vi "XL320_Configure Baud Rate.vi"(8 "error in (no error)":errorcluster, 9 "Baud rate (1,000,000 bps)":T1=3 items=["9600 bps", "57600 bps", "115200 bps", "1,000,000 bps"], 10 "Motor ID (0)":u8, 11 "VISA resource name":refnum<visa-resource-name>) -> (0 "error out":errorcluster, 3 "VISA resource name out":refnum<visa-resource-name>)   [LabVIEW 2017, in "Dynamixel XL320.lvlib"]
doc: "Sets the motor's baud rate. The motor will automatically \"reboot\" and respond to commands sent using the new baud rate."
uses:
  <instrlib>/Dynamixel XL320 (Drivers instrument)/Dynamixel XL320.lvlib
  <instrlib>/Dynamixel XL320 (Drivers instrument)/Public/Motor Operation/Low Level/XL320_Baud Setting.ctl
panel:
  # "Ghislain REMY, IUT de Cachan, 2015 December 2015"
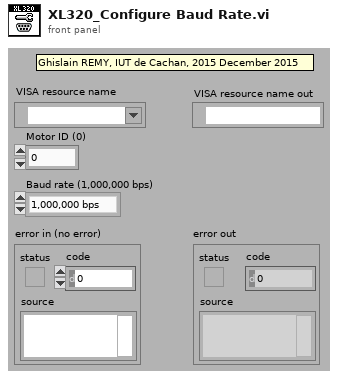
[diagram p1: front panel]
types:
  T1 = typedef "Dynamixel XL320.lvlib/XL320_Baud Setting.ctl" = u8
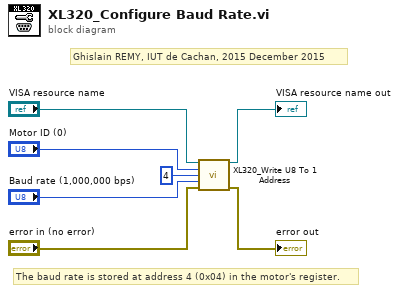
[diagram p0: block diagram]
diagram:
  # "Ghislain REMY, IUT de Cachan, 2015 December 2015"
  # "The baud rate is stored at address 4 (0x04) in the motor's register."
  n1 = call <instrlib>:"XL320_Write U8 To 1 Address.vi"("VISA resource name"="VISA resource name", "Motor ID (0)"="Motor ID (0)", "Address number (0)"=u16 4 ("Address"), "Parameter (0)"="Baud rate (1,000,000 bps)", "error in (no error)"="error in (no error)") -> ("VISA resource name out"=→"VISA resource name out":refnum<visa-resource-name>, "error out"=→"error out":errorcluster)  [unwired: 9 in]
